vi "Legend Initialize.vi"(6 "Control Ref Cluster":T1, 8 "error in (no error)":errorcluster, 10 "XY Plot Width":u32, 11 "3D Plot.lvclass":refnum<class "3D Plot.lvclass">) -> (0 "error out":errorcluster)   [LabVIEW 2020, in "3D Plot.lvclass"]
uses:
  3D Plot.lvclass
  3DMathPlot Ctrl Act Cluster.ctl
  3DMathPlot State Class.ctl
  3D Plot.lvclass/3D Plot.ctl
  NI_Math Plot Private Lib.lvlib
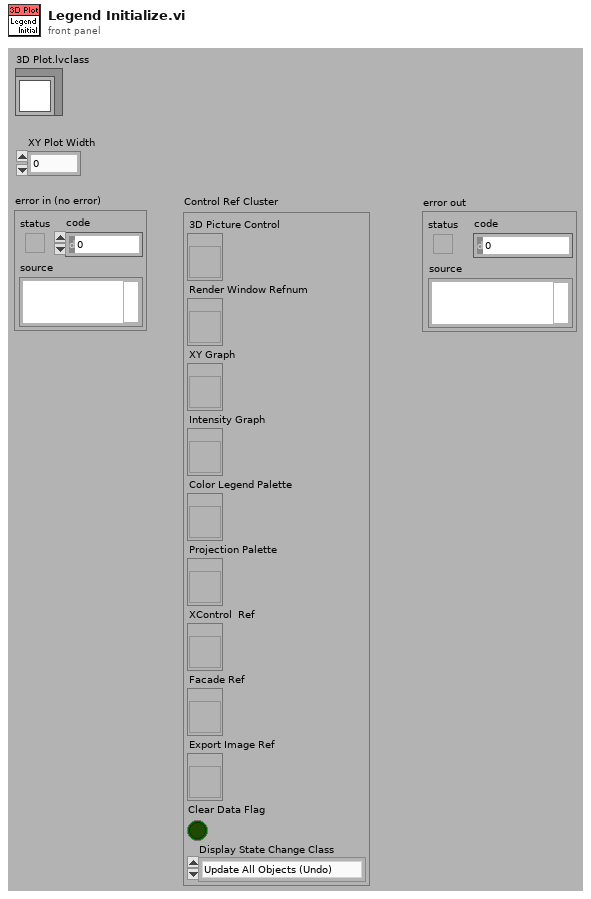
[diagram p1: front panel]
types:
  T1 = typedef "3DMathPlot Ctrl Act Cluster.ctl" = cluster{"3D Picture Control":refnum<vi>, "Render Window Refnum":refnum<vi>, "XY Graph":refnum<vi>, "Intensity Graph":refnum<vi>, "Color Legend Palette":refnum<vi>, "Projection Palette":refnum<vi>, "XControl  Ref":refnum<vi>, "Facade Ref":refnum<vi>, "Export Image Ref":refnum<vi>, "Clear Data Flag":bool, "Display State Change Class":T2}
  T2 = typedef "3DMathPlot State Class.ctl" = enum16{"Update All Objects (Undo)", "Update Light Object Only", "Update Axis Object Only", "Update Plot Object Only", "Update Cursor Object Only", "Update Axis Plot Cursor Objects", "No Update"}
  T3 = enum32{"Towards X-Y Plane", "Towards X-Z Plane", "Towards Y-Z Plane", "User Defined"}
  T4 = typedef "LVPositionTypeDef.ctl" = cluster{"Left":i32, "Top":i32}
  T5 = typedef "LVRectTypeDef.ctl" = cluster{"Left":i16, "Top":i16, "Right":i16, "Bottom":i16}
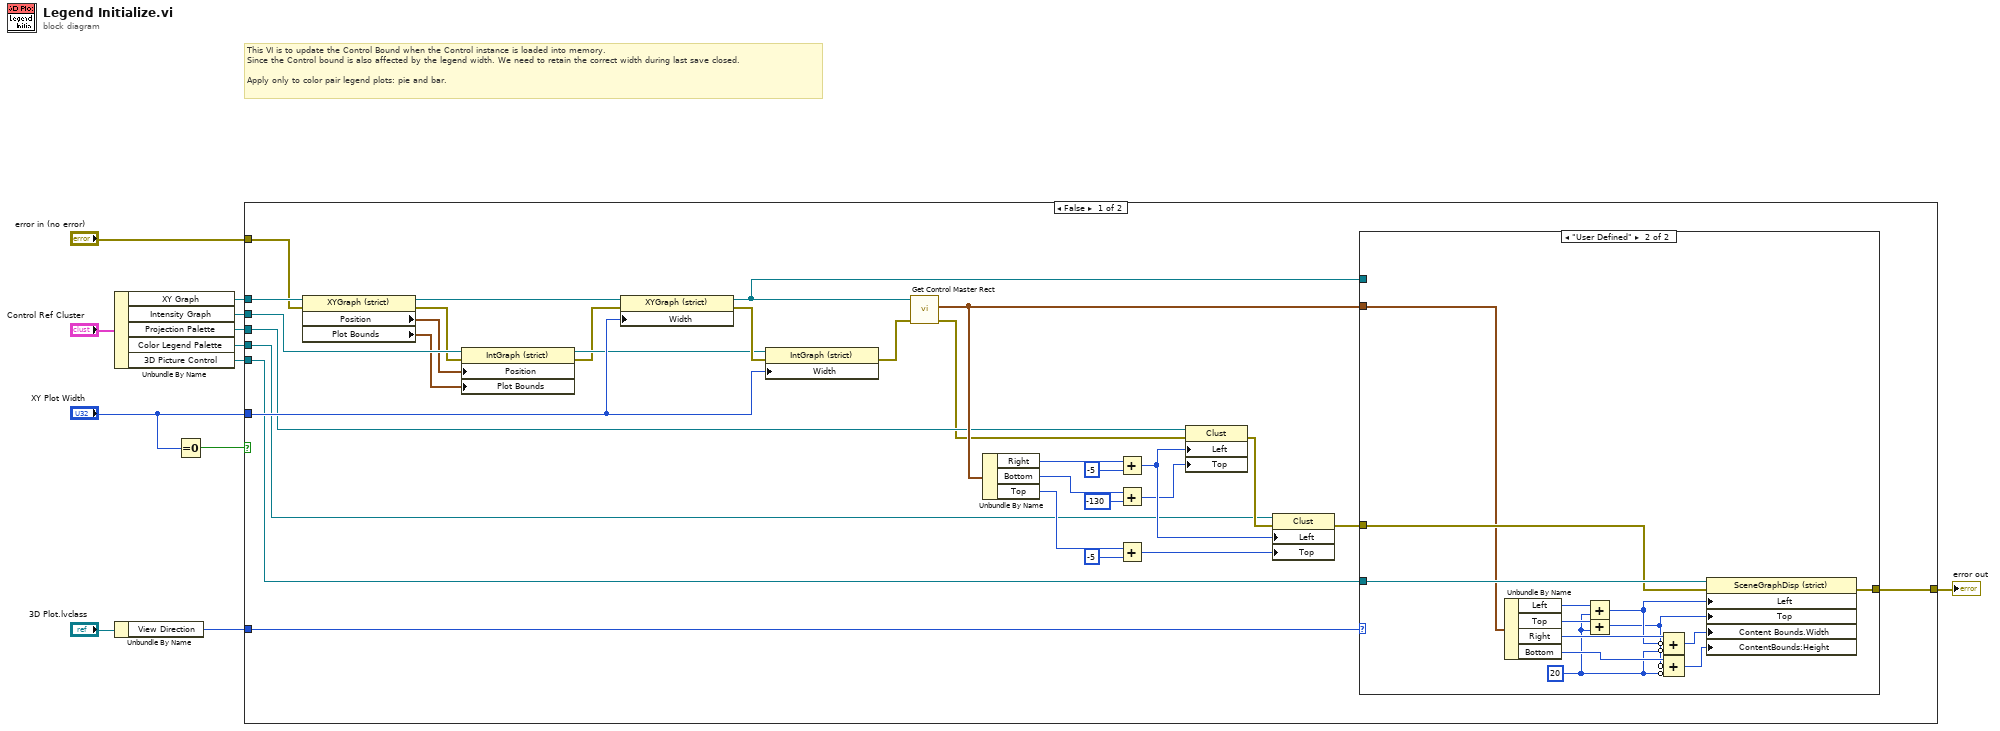
[diagram p0: block diagram]
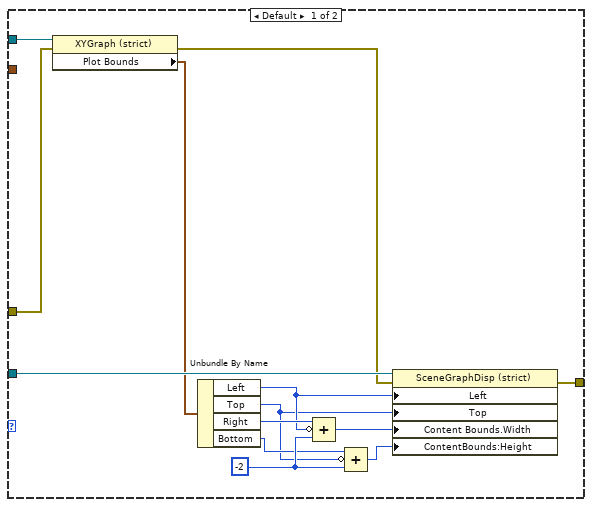
[diagram p2: hidden frame]
diagram:
  # "This VI is to update the Control Bound when the Control instance is loaded into memory.\nSince the Control bound is also affected by the legend width. We need to retain the correct width during last save closed.\n\nApply only to color pair legend plots: pie and bar."
  n1 = Unbundle By Name("Control Ref Cluster") -> ("XY Graph"=w8:refnum<vi>, "Intensity Graph"=w7:refnum<vi>, "Projection Palette"=w4:refnum<vi>, "Color Legend Palette"=w3:refnum<vi>, "3D Picture Control"=w5:refnum<vi>)
  n2 = Unbundle By Name("3D Plot.lvclass") -> ("View Direction"=w1:T3)
  n3 = Equal To 0?(x="XY Plot Width") -> (x = 0?=w10:bool)
  n4 = case shown="False" w10 {
    tunnel: "error in (no error)" -> [w21 w70]
    tunnel: [w30 w70] -> w11
    tunnel: "XY Plot Width" -> [w29 _]
    tunnel: w8 -> [w27 _]
    tunnel: w7 -> [w25 _]
    tunnel: w5 -> [w18 _]
    tunnel: w4 -> [w17 _]
    tunnel: w3 -> [w16 _]
    tunnel: w1 -> [w13 _]
    frame False {
      n5 = property on="Property Node" class="XYGraph (strict)"(reference=w27, error in=w21) -> (reference out=w26:refnum<vi>, error out=w20:errorcluster, "Position"=w23:T4, "Plot Bounds"=w22:T5)
      n6 = property on="Property Node" class="IntGraph (strict)"(reference=w25, error in=w20, "Position"=w23, "Plot Bounds"=w22) -> (reference out=w24:refnum<vi>, error out=w19:errorcluster)
      n7 = property class="XYGraph (strict)"(reference=w26, error in=w19, "Width"=w29) -> (reference out=w32:refnum<vi>, error out=w28:errorcluster)
      n8 = property class="IntGraph (strict)"(reference=w24, error in=w28, "Width"=w29) -> (error out=w15:errorcluster)  [unwired: 1 out]
      n9 = call "Get Control Master Rect.vi"("error in (no error)"=w15, "reference"=w32) -> ("error out"=w14:errorcluster, "Master Bounds Rect"=w33:T5)  [unwired: 8 out]
      n10 = Unbundle By Name(w33) -> ("Right"=w41:i16, "Bottom"=w35:i16, "Top"=w42:i16)
      n11 = Add(x=w41, y=i16 -5) -> (x+y=w43:i16)
      n12 = Add(x=w35, y=i16 -130) -> (x+y=w40:i16)
      n13 = Add(x=w42, y=i16 -5) -> (x+y=w38:i16)
      n14 = property on="Property Node" class="Clust"(reference=w17, error in=w14, "Left"=w43, "Top"=w40) -> (error out=w34:errorcluster)  [unwired: 1 out]
      n15 = property on="Property Node" class="Clust"(reference=w16, error in=w34, "Left"=w43, "Top"=w38) -> (error out=w31:errorcluster)  [unwired: 1 out]
      n16 = case shown="\"User Defined\"" w13 {
        tunnel: w18 -> [w56 w65]
        tunnel: w32 -> [w55 _]
        tunnel: w31 -> [w53 w58]
        tunnel: [w52 w60] -> w30
        tunnel: w33 -> [_ w57]
        frame Default {
          w51 = i16 -2
          n17 = property on="Property Node" class="XYGraph (strict)"(reference=w55, error in=w53) -> (error out=w54:errorcluster, "Plot Bounds"=w48:T5)  [unwired: 1 out]
          n18 = Unbundle By Name(w48) -> ("Left"=w47:i16, "Top"=w46:i16, "Right"=w49:i16, "Bottom"=w50:i16)
          n19 = Compound Arithmetic op=ADD(w49, invert w47, w51) -> (w45:i16)
          n20 = Compound Arithmetic op=ADD(w50, invert w46, w51) -> (w44:i16)
          n21 = property class="SceneGraphDisp (strict)"(reference=w56, error in=w54, "Left"=w47, "Top"=w46, "Content Bounds.Width"=w45, "ContentBounds:Height"=w44) -> (error out=w52:errorcluster)  [unwired: 1 out]
        }
        frame "User Defined" {
          w59 = i16 20 ("y")
          n22 = Unbundle By Name(w57) -> ("Left"=w67:i16, "Top"=w68:i16, "Right"=w66:i16, "Bottom"=w69:i16)
          n23 = Add(x=w67, y=w59) -> (x+y=w64:i16)
          n24 = Add(x=w68, y=w59) -> (x+y=w63:i16)
          n25 = Compound Arithmetic op=ADD(w66, invert w64, invert w59) -> (w62:i16)
          n26 = Compound Arithmetic op=ADD(w69, invert w63, invert w59) -> (w61:i16)
          n27 = property class="SceneGraphDisp (strict)"(reference=w65, error in=w58, "Left"=w64, "Top"=w63, "Content Bounds.Width"=w62, "ContentBounds:Height"=w61) -> (error out=w60:errorcluster)  [unwired: 1 out]
        }
      }
    }
    frame True {
    }
  }
  "error out" <- w11
